vi "New.vi"(6 "Configuration":string, 7 "Class Manager Reference":refnum<data-value>, 8 "error in (no error)":errorcluster, 10 "Name":string, 11 "Child Class in":refnum<class "Example Application.lvclass">) -> (0 "error out":errorcluster, 3 "Child Class out":refnum<class "Example Application.lvclass">)   [LabVIEW 2015, in "Example Application.lvlib" / "Example Application.lvclass"]
uses:
  Example Application.lvclass
  <vilib>/Cree, Inc/Cree Test Framework/Classes/Class Register/Class Register.lvclass
  CBTF Modules/Classes/Application/Class/Application.lvclass
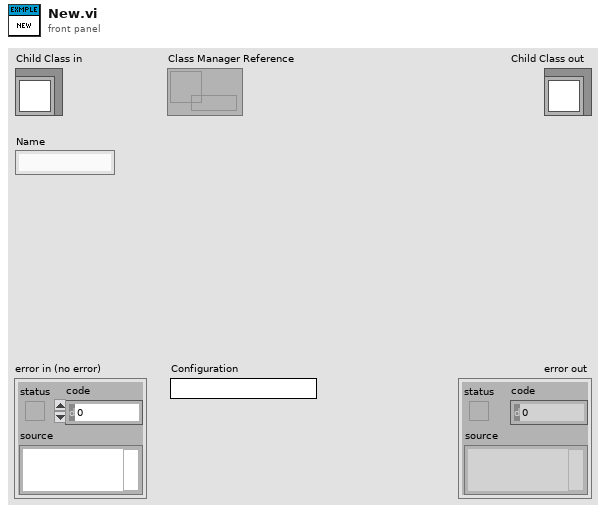
[diagram p1: front panel]
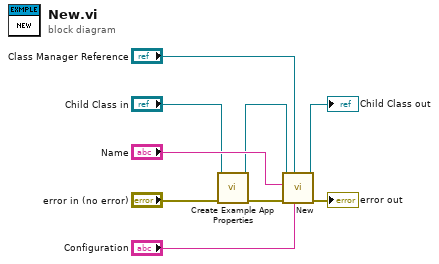
[diagram p0: block diagram]
diagram:
  n1 = call "Create Example App Properties.vi"("error in (no error)"="error in (no error)", "Acrobat Template in"="Child Class in") -> ("error out"=w3:errorcluster, "Acrobat Template out"=w1:refnum<class "Example Application.lvclass">)  [unwired: 8 in]
  n2 = call-parent "New.vi"("Configuration"="Configuration", "Class Manager Reference"="Class Manager Reference", "error in (no error)"=w3, "Name"="Name", "Child Class in"=w1) -> ("error out"=→"error out":errorcluster, "Child Class out"=→"Child Class out":refnum<class "Example Application.lvclass">)  [unwired: 5 in]
